vi "arm-execute-sim.vi"   [LabVIEW 2020]
uses:
  RobotCode/Arm/ArmGlobal.vi
  RobotCode/Human/HumanGlobal.vi
  arm-sim-globals.vi
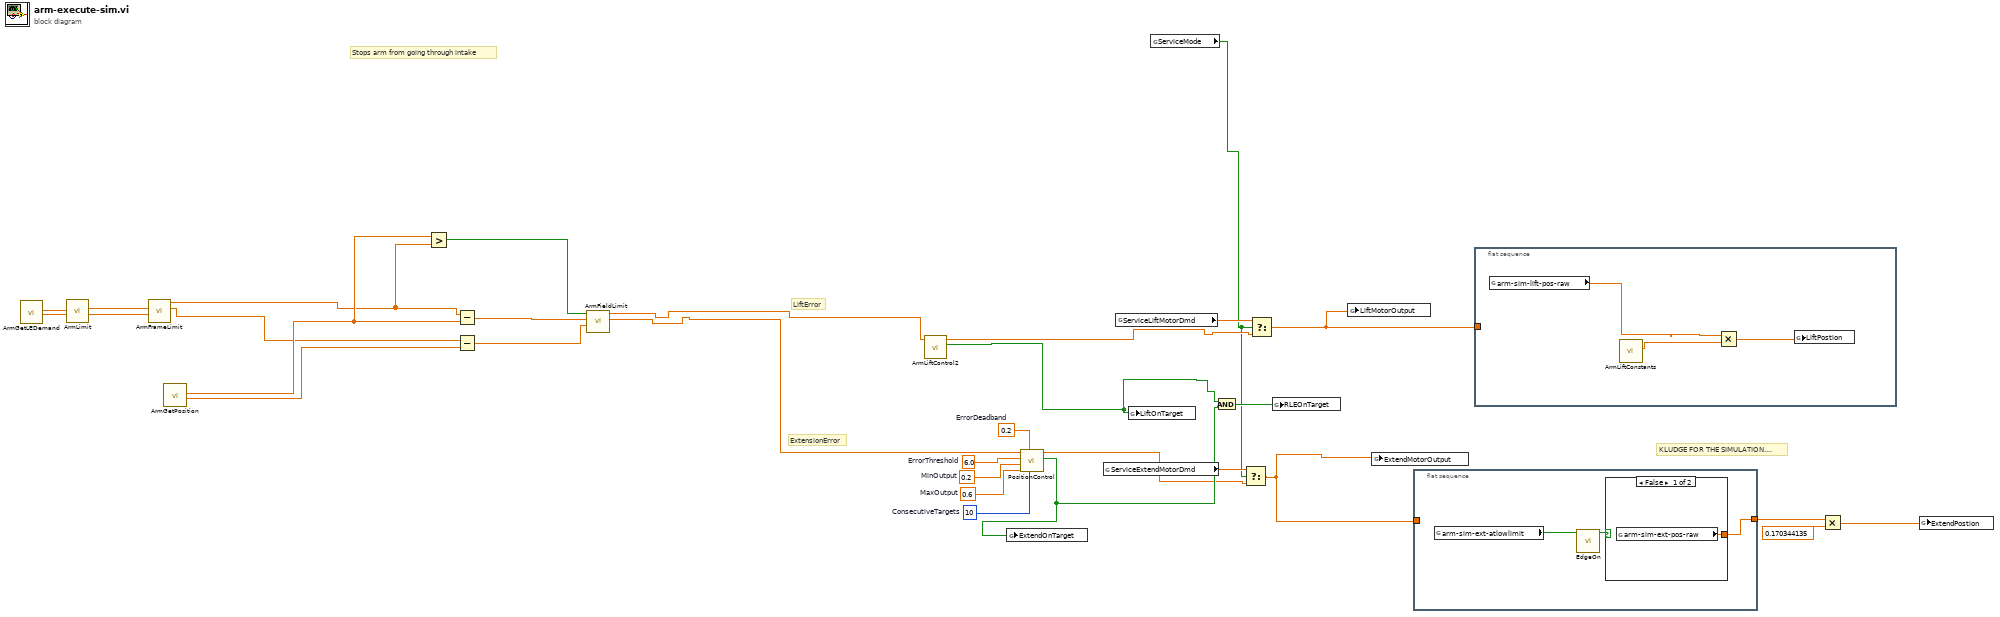
[diagram p0: block diagram]
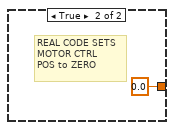
[diagram p2: hidden frame]
diagram:
  w27 = 10  # ConsecutiveTargets
  w28 = 0.6  # MaxOutput
  w29 = 0.2  # MinOutput
  w30 = 6.0  # ErrorThreshold
  w31 = 0.2  # ErrorDeadband
  # "KLUDGE FOR THE SIMULATION...."
  # "Stops arm from going through intake"
  # "ExtensionError"
  # "LiftError"
  n1 = call "ArmGetLEDemand.vi"() -> ("ExtendPositonDemand(in)"=w22:dbl, "LiftPositionDemand(d)"=w23:dbl)  [unwired: 10 in]
  n2 = call "ArmLimit.vi"("Extend"=w22, "Lift"=w23) -> ("Extend"=w6:dbl, "Lift"=w7:dbl)  [unwired: 8 in]
  n3 = call "ArmFrameLimit.vi"("Extend Setpoint"=w6, "Lift Setpoint"=w7) -> ("Extend Position"=w4:dbl, "Lift Setpoint"=w5:dbl)  [unwired: 8 in]
  n4 = call "ArmGetPosition.vi"() -> ("ExtendPostion"=w11:dbl, "LiftPostion"=w12:dbl)  [unwired: 10 in]
  n5 = Greater?(x=w12, y=w5) -> (0:w10:bool)
  n6 = Subtract(x=w5, y=w12) -> (x-y=w13:dbl)
  n7 = Subtract(x=w4, y=w11) -> (x-y=w14:dbl)
  n8 = call "ArmFieldLimit.vi"("Extend Error"=w14, "Lift Error"=w13, "Going Down?"=w10) -> ("Extend Error"=w8:dbl, "Lift Error"=w9:dbl)  [unwired: 7 in]
  n9 = call "ArmLiftControl2.vi"("erronIn(d)"=w9) -> ("OnTarget"=w15:bool, "motorOutput"=w19:dbl)  [unwired: 9 in]
  n10 = call "PositionControl.vi"("ConsecutiveTargets"=w27, "ErrorDeadband"=w31, "MaxOutput"=w28, "MinOutput"=w29, "ErrorThreshold"=w30, "Error"=w8) -> ("OnTarget"=w26:bool, "OutputValue"=w17:dbl)  [unwired: 3 in, 1 out]
  n11 = global write "ArmGlobal.vi" "ExtendOnTarget"(w26) -> ()
  n12 = global read "HumanGlobal.vi" "ServiceExtendMotorDmd"() -> (w18:dbl)
  n13 = global read "HumanGlobal.vi" "ServiceLiftMotorDmd"() -> (w20:dbl)
  n14 = global write "ArmGlobal.vi" "LiftOnTarget"(w15) -> ()
  n15 = global read "HumanGlobal.vi" "ServiceMode"() -> (w16:bool)
  n16 = And(x=w15, y=w26) -> (x .and. y?=w25:bool)
  n17 = Select(t=w18, s=w16, f=w17) -> (s? t:f=w2:dbl)
  n18 = Select(t=w20, s=w16, f=w19) -> (s? t:f=w1:dbl)
  n19 = global write "ArmGlobal.vi" "RLEOnTarget"(w25) -> ()
  n20 = global write "ArmGlobal.vi" "LiftMotorOutput"(w1) -> ()
  n21 = global write "ArmGlobal.vi" "ExtendMotorOutput"(w2) -> ()
  n22 = flat-sequence {
    tunnel: [w33] -> w3
    tunnel: w2 -> [_]
    frame #0 {
      n23 = global read "arm-sim-globals.vi" "arm-sim-ext-atlowlimit"() -> (w32:bool)
      n24 = call "EdgeOn.vi"("Current State"=w32) -> ("Edge On Found"=w34:bool)  [unwired: 10 in]
      n25 = case shown="False" w34 {
        tunnel: [w35 0.0 ("arm-sim-ext-pos-raw")] -> w33
        frame False {
          n26 = global read "arm-sim-globals.vi" "arm-sim-ext-pos-raw"() -> (w35:dbl)
        }
        frame True {
          # "REAL CODE SETS\nMOTOR CTRL\nPOS to ZERO"
        }
      }
    }
  }
  n27 = flat-sequence {
    tunnel: w1 -> [_]
    frame #0 {
      n28 = global read "arm-sim-globals.vi" "arm-sim-lift-pos-raw"() -> (w37:dbl)
      n29 = call "ArmLiftConstants.vi"() -> ("LiftConversionFactor"=w38:dbl)  [unwired: 9 in, 2 out]
      n30 = Multiply(x=w37, y=w38) -> (x*y=w39:dbl)
      n31 = global write "ArmGlobal.vi" "LiftPostion"(w39) -> ()
    }
  }
  n32 = Multiply(x=w3, y=0.170344135) -> (x*y=w21:dbl)
  n33 = global write "ArmGlobal.vi" "ExtendPostion"(w21) -> ()
